vi "변수.vi"() -> ()   [LabVIEW 2014]
panel:
  out "웨이브폼 차트 2":dbl(graph) caption="웨이브폼 차트"
  out "웨이브폼 차트":dbl(graph)
  in  "정지":bool
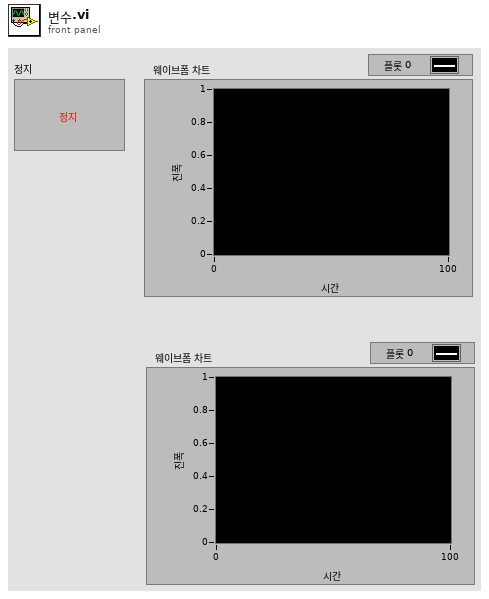
[diagram p1: front panel]
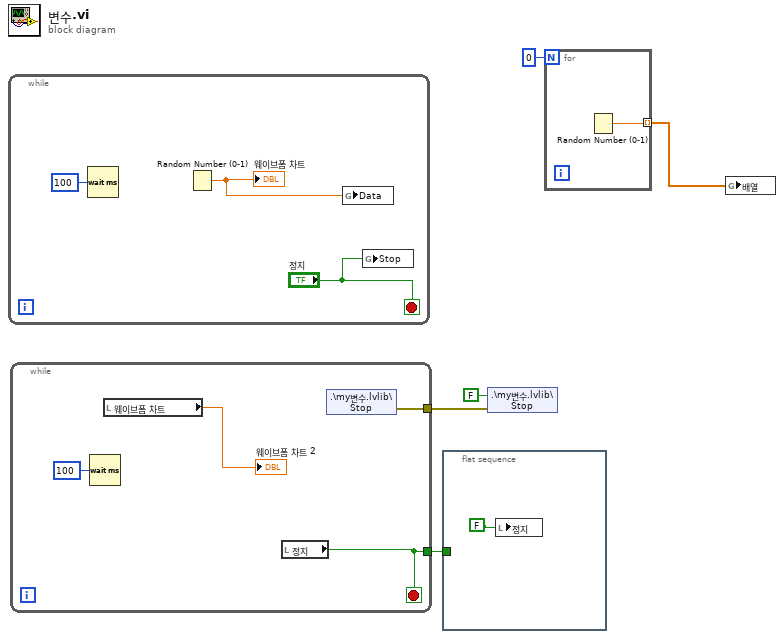
[diagram p0: block diagram]
diagram:
  n1 = while {
    stop <- "정지" stop-if-true
    n2 = Wait (ms)(milliseconds to wait=u32 100 ("대기 시간(ms)")) -> ()  [unwired: 1 out]
    n3 = Random Number (0-1)() -> (number: 0 to 1=w7:dbl)
    "웨이브폼 차트" <- w7
    n4 = global write "my글로벌.vi" "Data"(w7) -> ()
    n5 = global write "my글로벌.vi" "Stop"("정지") -> ()
  }
  n6 = while {
    tunnel: [w10] -> w5
    tunnel: [w9] -> w3
    stop <- w10 stop-if-true
    n7 = Wait (ms)(milliseconds to wait=u32 100 ("대기 시간(ms)")) -> ()  [unwired: 1 out]
    n8 = local read "웨이브폼 차트"() -> (→"웨이브폼 차트 2":dbl)
    n9 = local read "정지"() -> (w10:bool)
    n10 = shared-variable ".\\my변수.lvlib\\Stop"() -> (error out=w9:errorcluster)  [unwired: 1 in, 1 out]
  }
  n11 = flat-sequence {
    tunnel: w5 -> [_]
    frame #0 {
      n12 = local write "정지"(FALSE) -> ()
    }
  }
  n13 = shared-variable ".\\my변수.lvlib\\Stop"(FALSE ("Stop"), error in=w3) -> ()  [unwired: 1 out]
  n14 = for {
    N: 0 -> [_]
    tunnel: [w14] -> w4 mode=indexing
    n15 = Random Number (0-1)() -> (number: 0 to 1=w14:dbl)
  }
  n16 = global write "배열 글로벌.vi" "배열"(w4) -> ()
